vi "Begin (Austen Adler's conflicted copy 2013-10-16).vi"(11 "Image Size":T1=enum."160x120") -> (0 "error out":errorcluster)   [LabVIEW 2012]
doc: "Called before other user functions, this VI is expected to open initial I/O refnums, load in file data, and do all program initialization. Notice that the <B>error out</B> terminal is simply used for data flow. Wiring it to other structures or subVIs ensures that this VI runs first."
uses:
  <vilib>/Rock Robotics/WPI/Camera/WPI_CameraImageSize.ctl
  <vilib>/Rock Robotics/SystemInterfaces/DIO/FPGA_DIOPWMChannel.ctl
  <vilib>/Rock Robotics/WPI/Camera/WPI_CameraWhite Balance Values.ctl
  <vilib>/Rock Robotics/WPI/Camera/WPI_CameraExposure Values.ctl
  <vilib>/Rock Robotics/WPI/Camera/WPI_CameraFrameRate.ctl
  <vilib>/Rock Robotics/WPI/SafetyOutput/WPI_SafetyOutputConfigMenu.ctl
  <vilib>/Rock Robotics/WPI/DriverStation/WPI_DriverStationRobotMode2.ctl
  <vilib>/Rock Robotics/WPI/Joystick/WPI_JoystickDeviceEnum.ctl
  <vilib>/Rock Robotics/SystemInterfaces/DIO/FPGA_DIOChannel.ctl
  <vilib>/Rock Robotics/SystemInterfaces/DIO/FPGA_DIORelayChannel.ctl
  <vilib>/Rock Robotics/WPI/Solenoid/WPI_SolenoidChannel.ctl
  <vilib>/Rock Robotics/SystemInterfaces/AI/FPGA_AIChannel.ctl
  Robot Global Data.vi
  <vilib>/Rock Robotics/WPI/RobotDrive/WPI_RobotDriveOpen4MotorWithTalon.vi
  <vilib>/Rock Robotics/WPI/MotorControl/WPI_MotorControlOpen Talon.vi
  <vilib>/Rock Robotics/WPI/Solenoid/WPI_SolenoidOpenDouble.vi
  <vilib>/Rock Robotics/WPI/Compressor/WPI_CompressorGetSetRefNum.vi
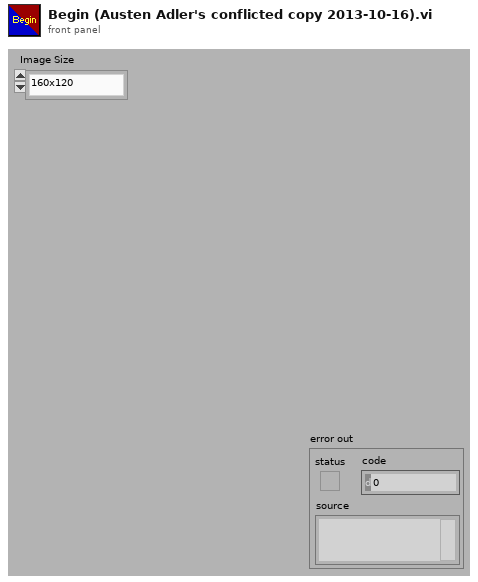
[diagram p1: front panel]
types:
  T1 = typedef "WPI_CameraImageSize.ctl" = enum16{"640x480", "320x240", "160x120"}
  T2 = typedef "WPI_SolenoidChannel.ctl" = enum8{"Solenoid 1", "Solenoid 2", "Solenoid 3", "Solenoid 4", "Solenoid 5", "Solenoid 6", "Solenoid 7", "Solenoid 8", "Invalid"}
  T3 = typedef "WPI_JoystickDeviceEnum.ctl" = enum16{"USB 1", "USB 2", "USB 3", "USB 4", "Kinect 1", "Kinect 2"}
  T4 = typedef "FPGA_DIOPWMChannel.ctl" = enum8{"PWM 1", "PWM 2", "PWM 3", "PWM 4", "PWM 5", "PWM 6", "PWM 7", "PWM 8", "PWM 9", "PWM 10", "Invalid"}
  T5 = typedef "FPGA_AIChannel.ctl" = enum8{"AI 1", "AI 2", "AI 3", "AI 4", "AI 5", "AI 6", "AI 7", "AI 8", "Invalid"}
  T6 = typedef "FPGA_DIOChannel.ctl" = enum8{"DIO 1", "DIO 2", "DIO 3", "DIO 4", "DIO 5", "DIO 6", "DIO 7", "DIO 8", "DIO 9", "DIO 10", "DIO 11", "DIO 12", "DIO 13", "DIO 14", "Invalid"}
  T7 = typedef "FPGA_DIORelayChannel.ctl" = enum8{"Relay 1", "Relay 2", "Relay 3", "Relay 4", "Relay 5", "Relay 6", "Relay 7", "Relay 8", "Invalid"}
  T8 = typedef "WPI_DriverStationRobotMode2.ctl" = enum16{"Autonomous Disabled", "Autonomous Enabled", "Teleop Disabled", "Teleop Enabled", "Timeout", "Finish", "Test Disabled", "Test Enabled"}
  T9 = typedef "WPI_SafetyOutputConfigMenu.ctl" = enum16{"Enable", "Disable"}
  T10 = typedef "WPI_CameraFrameRate.ctl" = u32
  T11 = typedef "WPI_CameraExposure Values.ctl" = enum16{"Auto", "Flicker-free 50 Hz", "Flicker-free 60 Hz", "Hold current"}
  T12 = typedef "WPI_CameraWhite Balance Values.ctl" = enum16{"Auto", "Fixed indoor", "Fixed outdoor 1", "Fixed outdoor 2", "Fixed fluorescent 1", "Fixed fluorescent 2", "Hold current"}
  T13 = typedef "WPI_CameraDevRef.ctl" = cluster{"Camera Address":string, "CameraStatus":errorcluster, "Acquire Image Notifier":refnum<notifier>}
  T14 = typedef "WPI_MotorControlDeviceRef.ctl" = cluster{"DeviceStatus":errorcluster, "Type":enum16{"PWM", "CAN"}, "PWM":cluster{"Digital Module":T15, "PWM Channel":T4, "DeadBand":T16}, "CAN":cluster{"Device Number":u8, "Control Mode":T17, "Semaphore":T18, "Max Vout":dbl}, "Invert":bool, "TransformRef":T19, "InvTransformRef":T19}
  T15 = typedef "FPGA_TypedefDigitalModule.ctl" = enum16{"Digital Module 1", "Digital Module 2"}
  T16 = typedef "WPI_PWMDeadband.ctl" = cluster{"Name":string, "maxPositivePwm":i32, "minPositivePwm":i32, "centerPwm":i32, "maxNegativePwm":i32, "minNegativePwm":i32, "angularRange":u16}
  T17 = typedef "WPI_CANJaguar_ControlMode.ctl" = enum8{"Percent VBus", "Current", "Speed", "Position", "Voltage"}
  T18 = typedef "Semaphore RefNum" = refnum<k1>
  T19 = typedef "WPI_PWMTransform_ConPane.ctl" = refnum<vi>
  T20 = typedef "WPI_RobotDriveDevRef.ctl" = cluster{"DevStatus":errorcluster, "Motors[]":T14[], "Square Inputs":bool, "Max Output":dbl, "Isochronous":bool}
  T21 = typedef "WPI_JoystickDevRef.ctl" = cluster{"Device":T3}
  T22 = typedef "WPI_SolenoidDevRef.ctl" = cluster{"DevStatus":errorcluster, "Solenoid Module":T23, "Forward Solenoid Channel":T2, "Reverse Solenoid Channel":T2}
  T23 = typedef "FPGA_TypedefSolenoidModule.ctl" = enum16{"Solenoid Module 1", "Solenoid Module 2"}
  T24 = typedef "WPI_AnalogChannelDevRef.ctl" = cluster{"DevStatus":errorcluster, "Analog Module":T25, "Analog Channel":T5}
  T25 = typedef "FPGA_TypedefAnalogModule.ctl" = enum16{"Analog Module 1", "Analog Module 2"}
  T26 = typedef "WPI_DigitalInputDevRef.ctl" = cluster{"DevStatus":errorcluster, "DIO Channel":T6, "Digital Module":T15}
  T27 = typedef "WPI_CompressorDevRef.ctl" = cluster{"DevStatus":errorcluster, "DigitalInputDevRef":T26, "RelayDevRef":T28}
  T28 = typedef "WPI_RelayDevRef.ctl" = cluster{"DevStatus":errorcluster, "Relay Channel":T7, "Digital Module":T15, "Relay Direction":T29}
  T29 = typedef "WPI_RelayDirection.ctl" = enum16{"Both directions", "Forward only", "Reverse only"}
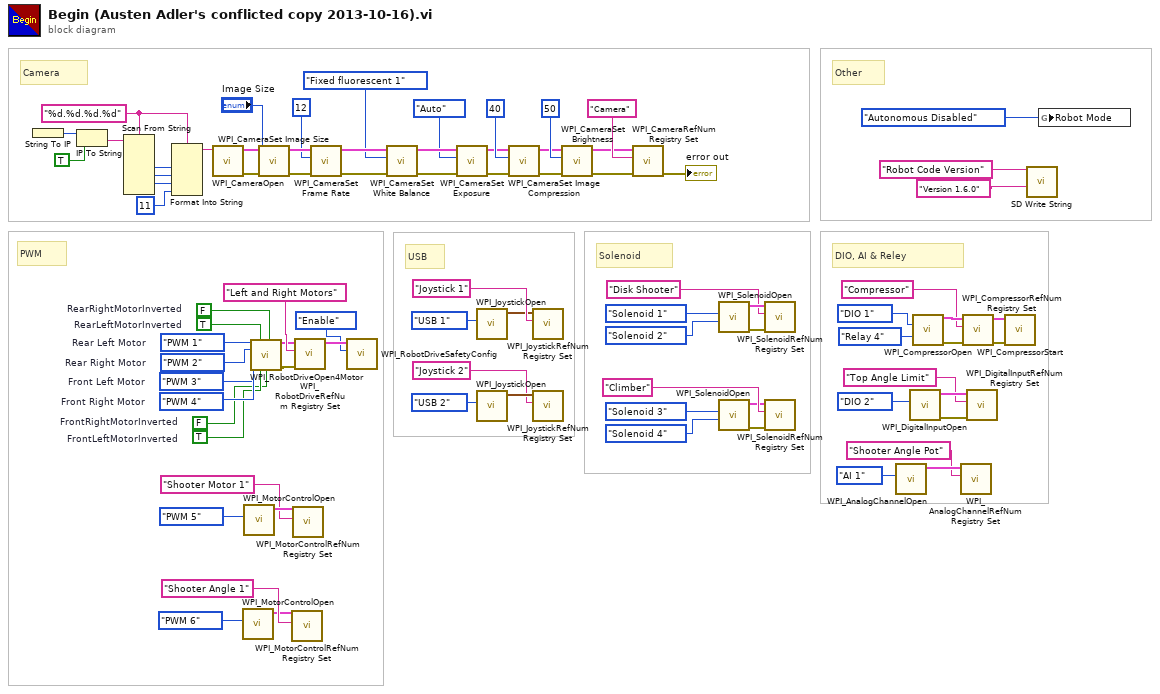
[diagram p0: block diagram]
diagram:
  w37 = TRUE  # FrontLeftMotorInverted
  w36 = FALSE  # FrontRightMotorInverted
  w39 = FPGA_DIOPWMChannel."PWM 4"  # Front Right Motor
  w38 = FPGA_DIOPWMChannel."PWM 3"  # Front Left Motor
  w54 = "%d.%d.%d.%d" ("format string")
  w40 = FPGA_DIOPWMChannel."PWM 2"  # Rear Right Motor
  w41 = FPGA_DIOPWMChannel."PWM 1"  # Rear Left Motor
  w43 = TRUE  # RearLeftMotorInverted
  w42 = FALSE  # RearRightMotorInverted
  # "Other"
  # "Camera"
  # "DIO, AI & Reley"
  # "PWM"
  # "Solenoid"
  # "USB"
  n1 = String To IP() -> (0:w61:u32)  [unwired: 1 in]
  n2 = IP To String(1:TRUE ("dot notation? (F)"), 2:w61) -> (0:w59:string)
  n3 = Scan From String(format string=w54, input string=w59) -> (output 1=w58:i32, output 2=w57:i32, output 3=w56:i32)  [unwired: 7 in, 3 out]
  n4 = Format Into String(format string=w54, w58, w57, w56, 11 ("Compression")) -> (resulting string=w50:string)  [unwired: 2 in, 1 out]
  n5 = call <vilib>:"WPI_CameraOpen.vi"("Camera Address"=w50) -> ("error out"=w73:errorcluster, "CameraDevRef"=w74:T13)  [unwired: 1 in, 8 out]
  n6 = call-poly <vilib>:"WPI_MotorControlOpen.vi"("PWM Channel"=FPGA_DIOPWMChannel."PWM 6") -> ("MotorControlDeviceRef"=w10:T14)  [unwired: 9 in, 1 out]
  n7 = call-poly <vilib>:"WPI_MotorControlOpen.vi"("PWM Channel"=FPGA_DIOPWMChannel."PWM 5") -> ("MotorControlDeviceRef"=w34:T14)  [unwired: 9 in, 1 out]
  n8 = call-poly <vilib>:"WPI_RobotDriveOpen4Motor.vi"("Rear Left Motor"=w41, "Rear Left Motor Inverted"=w43, "Rear Right Motor Inverted"=w42, "Rear Right Motor"=w40, "Front Left Motor"=w38, "Front Right Motor"=w39, "Front Left Motor Inverted"=w37, "Front Right Motor Inverted"=w36) -> ("RobotDriveDevRef"=w44:T20, "error out"=w45:errorcluster)  [unwired: 6 in]
  n9 = call <vilib>:"WPI_CameraSet Image Size.vi"("error in (no error)"=w73, "Image Size"="Image Size", "CameraDevRef"=w74) -> ("error out"=w72:errorcluster, "CameraDevRef Out"=w75:T13)  [unwired: 7 out]
  n10 = call <vilib>:"WPI_MotorControlRefNum Registry Set.vi"("refnum name"="Shooter Angle 1", "MotorControlDevRef"=w10) -> ()  [unwired: 8 in, 2 out]
  n11 = call <vilib>:"WPI_MotorControlRefNum Registry Set.vi"("refnum name"="Shooter Motor 1", "MotorControlDevRef"=w34) -> ()  [unwired: 8 in, 2 out]
  n12 = call <vilib>:"WPI_RobotDriveRefNum Registry Set.vi"("error in (no error)"=w45, "refnum name"="Left and Right Motors", "RobotDriveDevRef"=w44) -> ("RobotDriveDevRef"=w53:T20)  [unwired: 8 out]
  n13 = call <vilib>:"WPI_CameraSet Frame Rate.vi"("error in (no error)"=w72, "Frame Rate (fps)"=T10 12, "CameraDevRef"=w75) -> ("error out"=w71:errorcluster, "CameraDevRef Out"=w77:T13)  [unwired: 7 out]
  n14 = call <vilib>:"WPI_RobotDriveSafetyConfig.vi"("mode"=WPI_SafetyOutputConfigMenu."Enable", "RobotDriveDevRef"=w53) -> ()  [unwired: 8 in, 2 out]
  n15 = call <vilib>:"WPI_CameraSet White Balance.vi"("error in (no error)"=w71, "White Balance"=WPI_CameraWhite_Balance_Values."Fixed fluorescent 1", "CameraDevRef"=w77) -> ("error out"=w70:errorcluster, "CameraDevRef Out"=w76:T13)  [unwired: 7 out]
  n16 = call <vilib>:"WPI_CameraSet Exposure.vi"("error in (no error)"=w70, "Exposure"=WPI_CameraExposure_Values."Auto", "CameraDevRef"=w76) -> ("error out"=w69:errorcluster, "CameraDevRef Out"=w79:T13)  [unwired: 7 out]
  n17 = call <vilib>:"WPI_JoystickOpen.vi"("JoystickDevice"=WPI_JoystickDeviceEnum."USB 1") -> ("JoystickDevRef"=w48:T21)  [unwired: 10 in]
  n18 = call <vilib>:"WPI_JoystickOpen.vi"("JoystickDevice"=WPI_JoystickDeviceEnum."USB 2") -> ("JoystickDevRef"=w7:T21)  [unwired: 10 in]
  n19 = call <vilib>:"WPI_CameraSet Image Compression.vi"("error in (no error)"=w69, "Compression"=40, "CameraDevRef"=w79) -> ("error out"=w68:errorcluster, "CameraDevRef Out"=w78:T13)  [unwired: 7 out]
  n20 = call <vilib>:"WPI_JoystickRefNum Registry Set.vi"("refnum name"="Joystick 1", "JoystickDevRef"=w48) -> ()  [unwired: 8 in, 2 out]
  n21 = call <vilib>:"WPI_JoystickRefNum Registry Set.vi"("refnum name"="Joystick 2", "JoystickDevRef"=w7) -> ()  [unwired: 8 in, 2 out]
  n22 = call <vilib>:"WPI_CameraSet Brightness.vi"("error in (no error)"=w68, "Brightness"=50, "CameraDevRef"=w78) -> ("error out"=w66:errorcluster, "CameraDevRef Out"=w67:T13)  [unwired: 7 out]
  n23 = call <vilib>:"WPI_CameraRefNum Registry Set.vi"("error in (no error)"=w66, "refnum name"="Camera", "CameraDevRef"=w67) -> ("error out"=→"error out":errorcluster)  [unwired: 8 out]
  n24 = call-poly <vilib>:"WPI_SolenoidOpen.vi"("Reverse Solenoid Channel"=WPI_SolenoidChannel."Solenoid 2" ("Forward Solenoid Channel"), "Forward Solenoid Channel"=WPI_SolenoidChannel."Solenoid 1" ("Solenoid Channel")) -> ("error out"=w24:errorcluster, "SolenoidDevRef"=w23:T22)  [unwired: 8 in]
  n25 = call-poly <vilib>:"WPI_SolenoidOpen.vi"("Reverse Solenoid Channel"=WPI_SolenoidChannel."Solenoid 4" ("Forward Solenoid Channel"), "Forward Solenoid Channel"=WPI_SolenoidChannel."Solenoid 3" ("Solenoid Channel")) -> ("error out"=w2:errorcluster, "SolenoidDevRef"=w3:T22)  [unwired: 8 in]
  n26 = call <vilib>:"WPI_SolenoidRefNum Registry Set.vi"("error in (no error)"=w24, "refnum name"="Disk Shooter", "SolenoidDevRef"=w23) -> ()  [unwired: 7 in, 2 out]
  n27 = call <vilib>:"WPI_SolenoidRefNum Registry Set.vi"("error in (no error)"=w2, "refnum name"="Climber", "SolenoidDevRef"=w3) -> ()  [unwired: 7 in, 2 out]
  n28 = call <vilib>:"WPI_AnalogChannelOpen.vi"("Analog Channel"=FPGA_AIChannel."AI 1") -> ("AIDeviceRef"=w14:T24)  [unwired: 9 in, 1 out]
  n29 = call <vilib>:"WPI_DigitalInputOpen.vi"("DIO Channel"=FPGA_DIOChannel."DIO 2") -> ("error out"=w20:errorcluster, "DigitalInputDevRef"=w19:T26)  [unwired: 9 in]
  n30 = call <vilib>:"WPI_CompressorOpen.vi"("Pressure Switch DIO Channel"=FPGA_DIOChannel."DIO 1", "Relay Channel"=FPGA_DIORelayChannel."Relay 4") -> ("CompressorDevRef"=w30:T27, "error out"=w27:errorcluster)  [unwired: 12 in]
  n31 = call <vilib>:"WPI_AnalogChannelRefNum Registry Set.vi"("refnum name"="Shooter Angle Pot", "AIDeviceRef"=w14) -> ()  [unwired: 8 in, 2 out]
  n32 = call <vilib>:"WPI_CompressorRefNum Registry Set.vi"("error in (no error)"=w27, "refnum name"="Compressor", "CompressorDevRef"=w30) -> ("error out"=w32:errorcluster, "CompressorDevRef"=w31:T27)  [unwired: 7 in]
  n33 = call <vilib>:"WPI_DigitalInputRefNum Registry Set.vi"("error in (no error)"=w20, "refnum name"="Top Angle Limit", "DigitalInputDevRef"=w19) -> ()  [unwired: 7 in, 2 out]
  n34 = call <vilib>:"WPI_CompressorStart.vi"("error in (no error)"=w32, "CompressorDevRef"=w31) -> ()  [unwired: 8 in, 2 out]
  n35 = call <vilib>:"SD Write String.vi"("String"="Version 1.6.0", "Name"="Robot Code Version") -> ()  [unwired: 8 in, 2 out]
  n36 = global write "Robot Global Data.vi" "Robot Mode"(WPI_DriverStationRobotMode2."Autonomous Disabled" ("Robot Mode")) -> ()
